vi "initialize editor node if needed.vi"(11 "editor node in":T1) -> (2 "engine":refnum<data-value>, 3 "editor node out":T1)   [LabVIEW 2013, in "tag bus processing plugin editor node.lvclass"]
uses:
  tag bus processing plugin editor node.lvclass
  <vilib>/CEF_TreeControl/Node/NodeRef.ctl
  <vilib>/CEF_TreeControl/Node/NISE_CEF_Node.lvclass
  Configuration Editor/Classes/Engine Parent/Engine Parent Editor Node.lvclass
  module/configuration/tag bus processing plugin module configuration.lvclass
  <vilib>/NI/Module Execution Interface/Engine Configuration/engine configuration.lvclass
  <vilib>/NI/Tag Bus/tag/Data Type.ctl
  <vilib>/NI/Tag Bus/tag/tag descriptor.lvclass/tag descriptor.ctl
  Configuration Editor/Classes/Engine Parent/read engine configuration.vi
  <vilib>/NI/Tag Bus/tag bus error generator.vi
  <vilib>/NI/Tag Bus/tag/validate default value.vi
  Configuration Editor/Classes/Engine Parent/write engine configuration.vi
  <vilib>/NI/Tag Bus/tag/tag descriptor.lvclass
  Configuration Editor/Classes/Module editor node/module editor node.lvclass
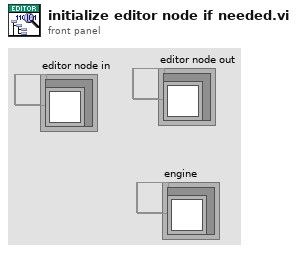
[diagram p1: front panel]
types:
  T1 = typedef "NISE_CEF_Node.lvclass/NodeRef.ctl" = refnum<data-value>
  T2 = typedef "tag bus.lvlib/tag descriptor.lvclass/Data Type.ctl" = enum16{"Double", "Single", "I64", "I32", "I16", "I8", "U64", "U32", "U16", "U8", "Boolean", "String", "Array of Double", "Array of Single", "Array of I64", "Array of I32", "Array of I16", "Array of I8", "Array of U64", "Array of U32", "Array of U16", "Array of U8", "Array of Boolean", "Array of String"}
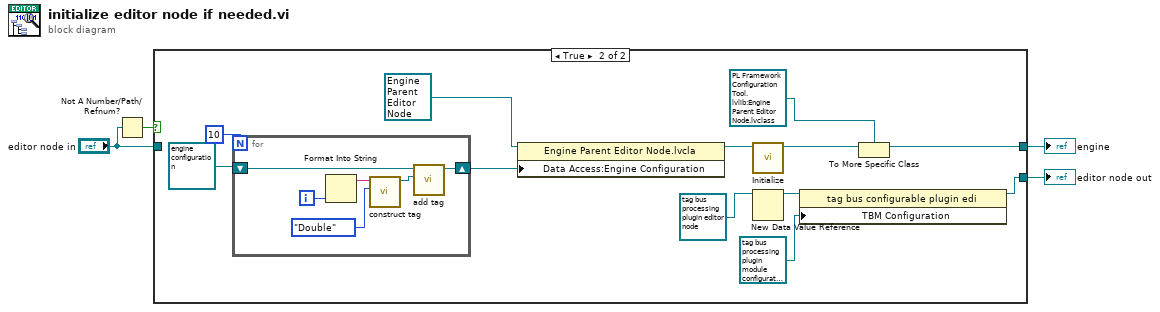
[diagram p0: block diagram]
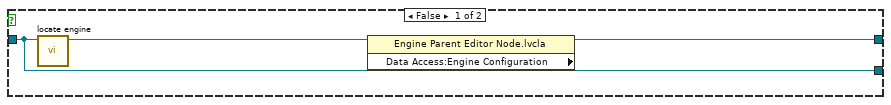
[diagram p2: hidden frame]
diagram:
  n1 = Not A Number/Path/Refnum?(number/path/refnum="editor node in") -> (NaN/Path/Refnum?=w1:bool)
  n2 = case shown="True" w1 {
    tunnel: "editor node in" -> [w6 _]
    tunnel: [w6 w19] -> w3
    tunnel: [w5 w17] -> w2
    frame False {
      n3 = call "locate engine.vi"("component"=w6) -> ("engine"=w7:refnum<data-value>)  [unwired: 9 in, 1 out]
      n4 = property class="Engine Parent Editor Node.lvcla" props=["Data Access:Engine Configuration"](reference=w7) -> (reference out=w5:refnum<data-value>)  [unwired: 1 in, 2 out]
    }
    frame True {
      n5 = for {
        N: 10 -> [_]
        shift-right: [w24] -> w8
        shift-left: refnum<class "engine configuration.lvclass"> refnum ("Engine Configuration") -> [w25]
        i -> [w22]
        n6 = Format Into String(w22) -> (resulting string=w21:string)  [unwired: 3 in, 1 out]
        n7 = call <vilib>:"construct tag.vi"("data type"=Data_Type."Double", "name"=w21) -> ("system tag out"=w23:refnum<class "tag descriptor.lvclass">)  [unwired: 8 in, 1 out]
        n8 = call <vilib>:"add tag.vi"("tag descriptor"=w23, "engine configuration in"=w25) -> ("engine configuration out"=w24:refnum<class "engine configuration.lvclass">)  [unwired: 8 in, 1 out]
      }
      n9 = property class="Engine Parent Editor Node.lvcla"(reference=refnum<class "Engine Parent Editor Node.lvclass"> refnum ("PL Framework Configuration Tool.lvlib:Engine Parent Editor Node.lvclass"), "Data Access:Engine Configuration"=w8) -> (reference out=w12:refnum<class "Engine Parent Editor Node.lvclass">)  [unwired: 1 in, 1 out]
      n10 = call-dynamic "Initialize.vi"("Engine in"=w12) -> ("data value reference"=w18:T1)  [unwired: 8 in, 2 out]
      n11 = New Data Value Reference(data value=refnum<class "tag bus processing plugin editor node.lvclass"> refnum ("tag bus configurable plugin editor node")) -> (data value reference=w15:refnum<data-value>)  [unwired: 1 in, 1 out]
      n12 = property class="tag bus configurable plugin edi"(reference=w15, "TBM Configuration"=refnum<class "tag bus processing plugin module configuration.lvclass"> refnum ("tag bus configurable plugin module configuration")) -> (reference out=w19:refnum<data-value>)  [unwired: 1 in, 1 out]
      n13 = To More Specific Class(target class=refnum<data-value> refnum ("data value reference"), reference=w18) -> (specific class reference=w17:refnum<data-value>)  [unwired: 1 in, 1 out]
    }
  }
  "editor node out" <- w3
  "engine" <- w2
